vi "STOP.vi"(10 "stop":bool, 11 "Select COM port":refnum<visa-resource-name>="COM3") -> (3 "False":bool)   [LabVIEW 2012]
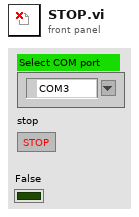
[diagram p1: front panel]
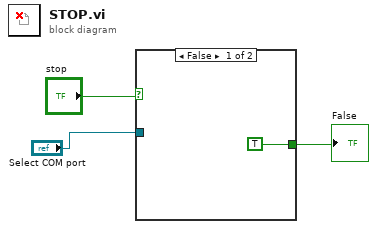
[diagram p0: block diagram]
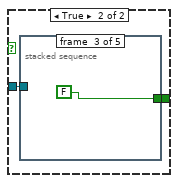
[diagram p2: hidden frame]
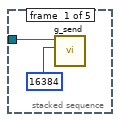
[diagram p3: hidden frame]
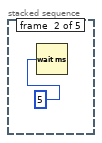
[diagram p4: hidden frame]
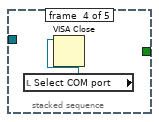
[diagram p5: hidden frame]
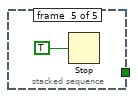
[diagram p6: hidden frame]
diagram:
  n1 = case shown="False" "stop" {
    tunnel: "Select COM port" -> [_ w6]
    tunnel: [TRUE w5] -> w1
    frame False {
    }
    frame True {
      n2 = stacked-sequence {
        tunnel: w6 -> [w7 _ _ _ _]
        tunnel: [_ _ FALSE _ _] -> w5
        frame #0 {
          n3 = call "g_send.vi"("Input buffer size"=16384, "USB Interface Name"=w7) -> ()  [unwired: 9 in, 1 out]
        }
        frame #1 {
          n4 = Wait (ms)(milliseconds to wait=5) -> ()  [unwired: 1 out]
        }
        frame #2 {
        }
        frame #3 {
          n5 = local read "Select COM port"() -> (w11:refnum<visa-resource-name>)
          n6 = VISA Close(VISA resource name=w11) -> ()  [unwired: 1 in, 1 out]
        }
        frame #4 {
          n7 = Stop(stop? (T)=TRUE ("Stop? (T)")) -> ()
        }
      }
    }
  }
  "False" <- w1
